vi "Digital Pulse Output.vi"() -> ()   [LabVIEW 2019]
uses:
  <vilib>/Utility/error.llb/DialogType.ctl
  <vilib>/DAQmx/configure/timing.llb/DAQmx Timing (Implicit).vi
  <vilib>/DAQmx/create/channels.llb/DAQmx Create Channel (CO-Pulse Generation-Frequency).vi
  <vilib>/DAQmx/read.llb/DAQmx Read (Counter 1D U32 1Chan NSamp).vi
  <vilib>/DAQmx/create/channels.llb/DAQmx Create Channel (CI-Count Edges).vi
panel:
  out "Waveform Chart":dynamicdata(graph)
  in  "stop (F) 2":bool caption="stop (F)"
  in  "stop (F)":bool
  in  "Stop":bool
  in  "counter":tag
  in  "counter 2":tag
  in  "Samples per Loop":i32=100
  in  "Stop 2":bool
  out "Data":u32[](array[numeric])
  in  "Duty Cycle":dbl=0.5 format="%.6f"
  in  "Frequency":dbl=1.0 format="%.6f"
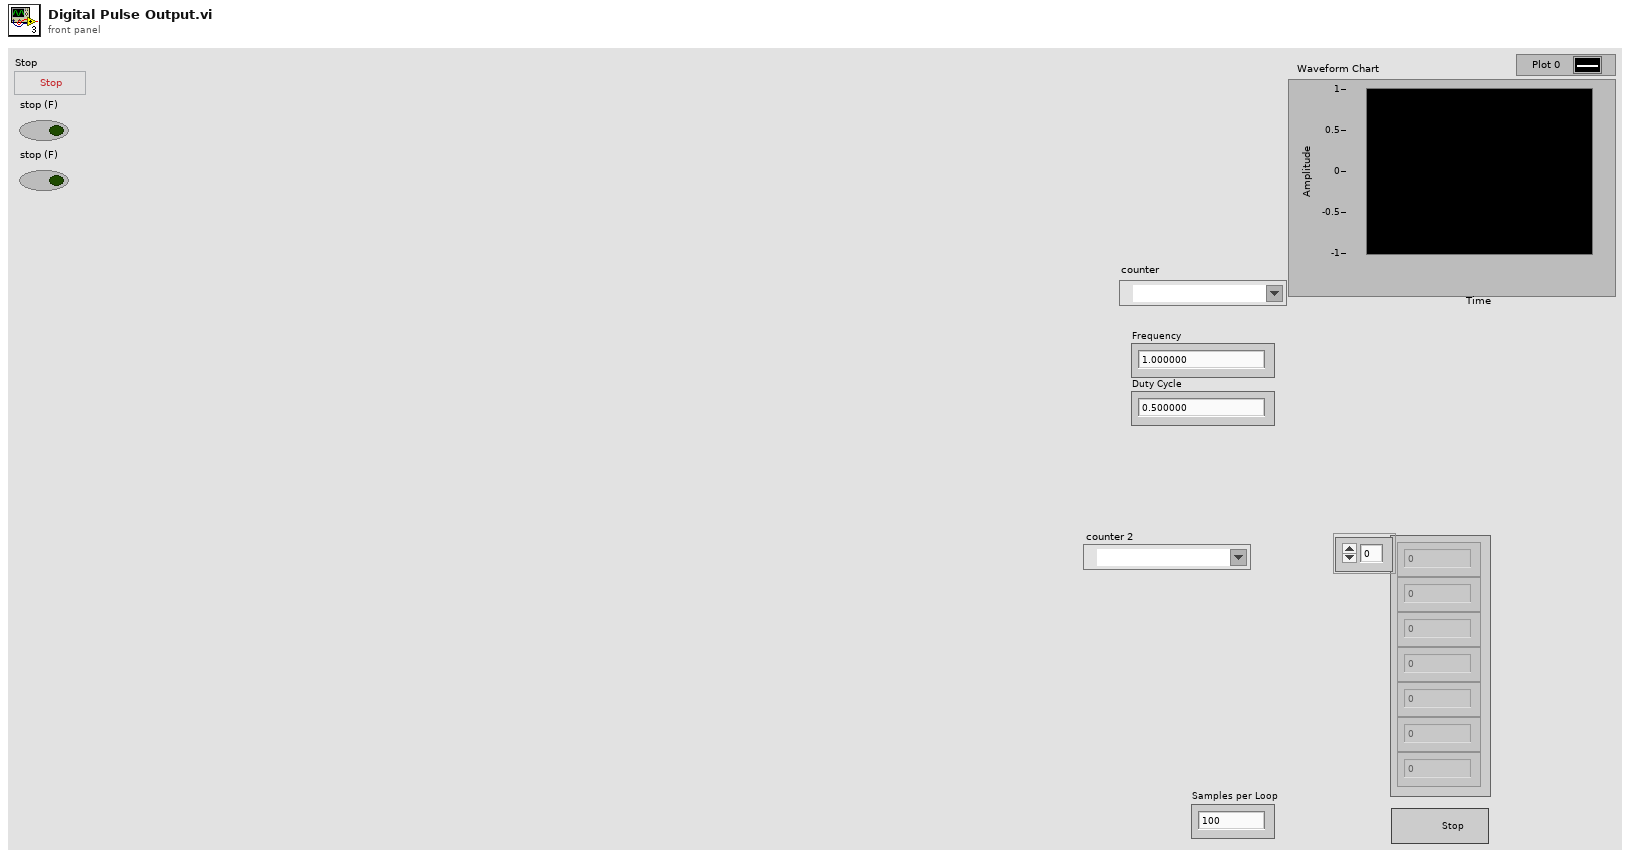
[diagram p1: front panel]
types:
  T1 = typedef "DialogType.ctl" = u16
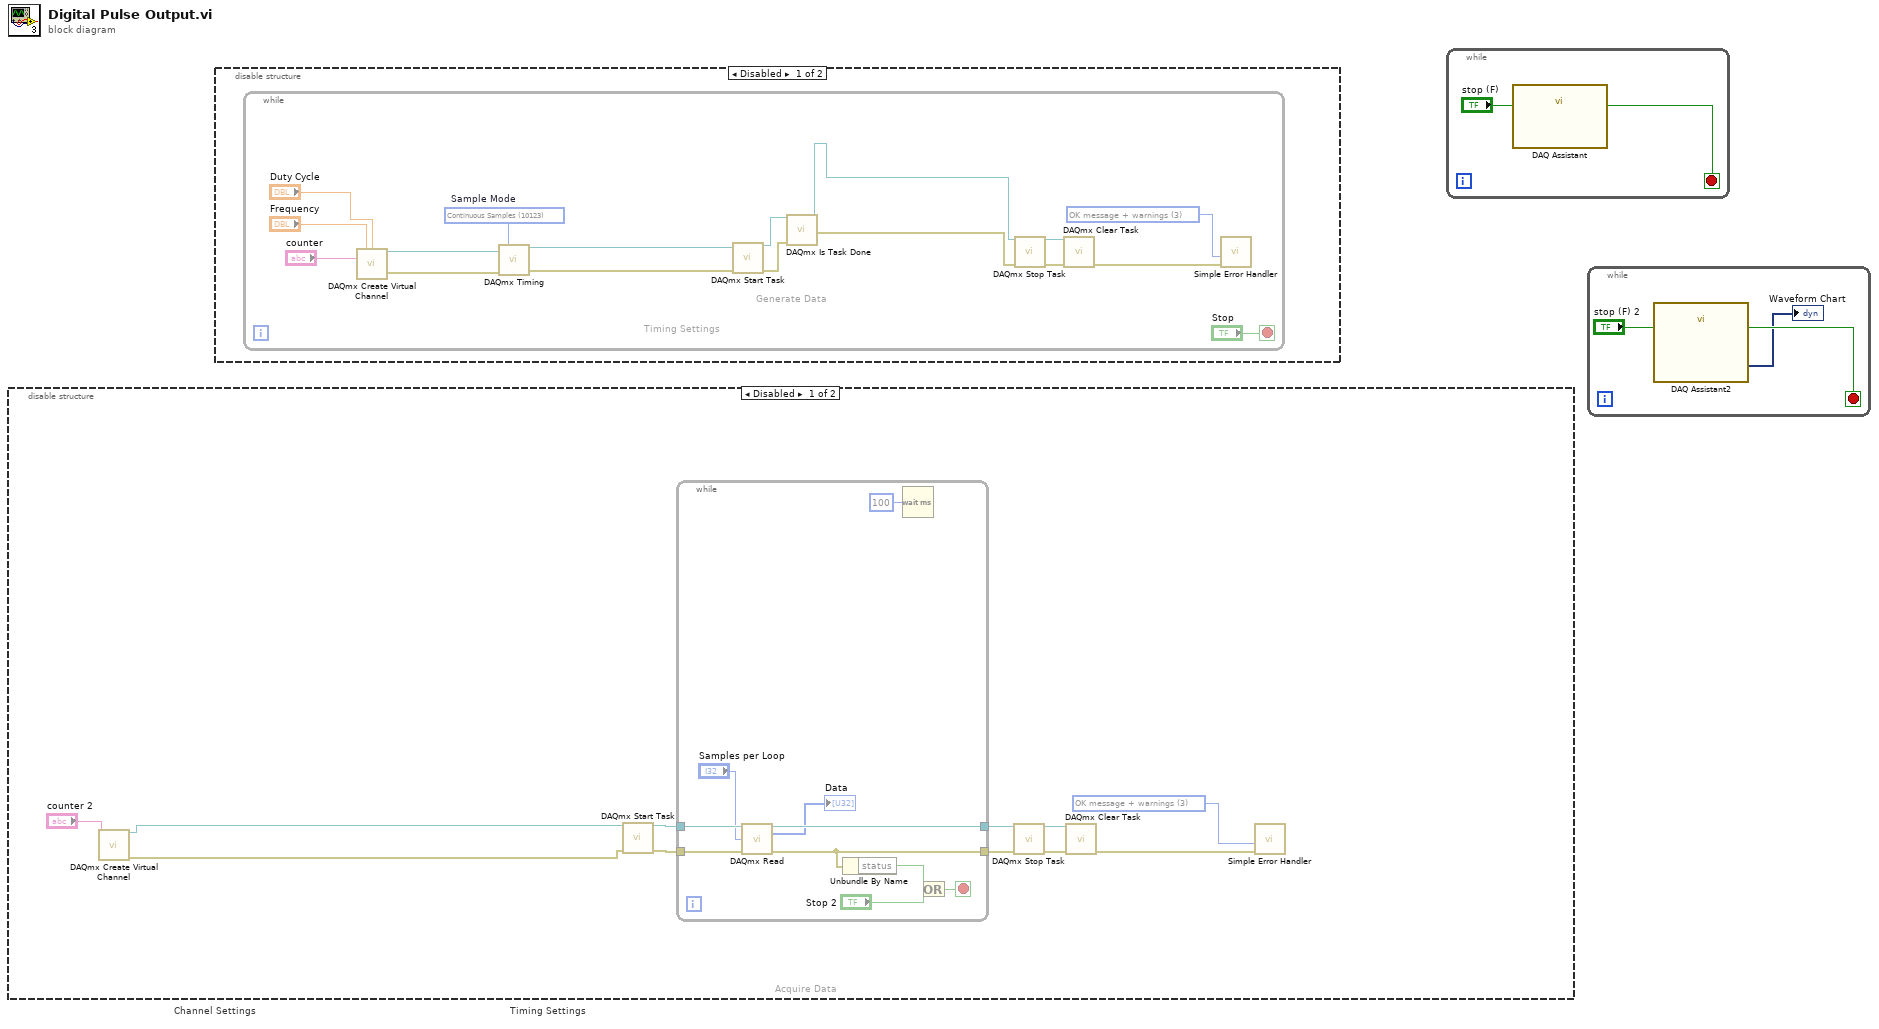
[diagram p0: block diagram]
diagram:
  # "Timing Settings"
  # "Channel Settings"
  n1 = disable-structure shown="Disabled" {
    frame Disabled {
      w4 = T1 3 items=["no dialog", "OK message", "continue or stop message", "OK message + warnings", "continue/stop + warnings"] ("type of dialog (OK msg:1)")
      # "Acquire Data"
      n2 = call-poly <vilib>:"DAQmx Create Virtual Channel.vi"("counter"="counter 2") -> ("task out"=w2:refnum<k21>, "error out"=w1:errorcluster)  [unwired: 13 in]
      n3 = call <vilib>:"DAQmx Start Task.vi"("task/channels in"=w2, "error in"=w1) -> ("task out"=w11:refnum<k21>, "error out"=w10:errorcluster)  [unwired: 12 in]
      n4 = while {
        tunnel: w11 -> [w21]
        tunnel: w10 -> [w20]
        tunnel: [w17] -> w7
        tunnel: [w18] -> w8
        stop <- w19 stop-if-true
        n5 = call-poly <vilib>:"DAQmx Read.vi"("task/channels in"=w21, "number of samples per channel"="Samples per Loop", "error in"=w20) -> ("task out"=w18:refnum<k21>, "data"=→"Data":u32[], "error out"=w17:errorcluster)  [unwired: 10 in]
        n6 = Unbundle By Name(w17) -> ("status"=w16:bool)
        n7 = Wait (ms)(milliseconds to wait=u32 100) -> ()  [unwired: 1 out]
        n8 = Or(x=w16, y="Stop 2") -> (x .or. y?=w19:bool)
      }
      n9 = call <vilib>:"DAQmx Stop Task.vi"("task/channels in"=w8, "error in"=w7) -> ("task out"=w5:refnum<k21>, "error out"=w6:errorcluster)  [unwired: 12 in]
      n10 = call <vilib>:"DAQmx Clear Task.vi"("task in"=w5, "error in"=w6) -> ("error out"=w9:errorcluster)  [unwired: 13 in]
      n11 = call <vilib>:"Simple Error Handler.vi"("type of dialog (OK msg:1)"=w4, "error in (no error)"=w9) -> ()  [unwired: 3 in, 5 out]
    }
    frame Enabled {
    }
  }
  n12 = disable-structure shown="Disabled" {
    frame Disabled {
      n13 = while {
        stop <- "Stop" stop-if-true
        w34 = T1 3 items=["no dialog", "OK message", "continue or stop message", "OK message + warnings", "continue/stop + warnings"] ("type of dialog (OK msg:1)")
        w38 = 10123 items=["Finite Samples"=10178, "Continuous Samples"=10123, "Hardware Timed Single Point"=12522]  # Sample Mode
        # "Generate Data"
        # "Timing Settings"
        n14 = call-poly <vilib>:"DAQmx Create Virtual Channel.vi"("frequency"="Frequency", "duty cycle"="Duty Cycle", "counter"="counter") -> ("task out"=w32:refnum<k21>, "error out"=w31:errorcluster)  [unwired: 11 in]
        n15 = call-poly <vilib>:"DAQmx Timing.vi"("task/channels in"=w32, "sample mode"=w38, "error in"=w31) -> ("task out"=w28:refnum<k21>, "error out"=w27:errorcluster)  [unwired: 11 in]
        n16 = call <vilib>:"DAQmx Start Task.vi"("task/channels in"=w28, "error in"=w27) -> ("task out"=w26:refnum<k21>, "error out"=w25:errorcluster)  [unwired: 12 in]
        n17 = call <vilib>:"DAQmx Is Task Done.vi"("task/channels in"=w26, "error in"=w25) -> ("task out"=w23:refnum<k21>, "error out"=w24:errorcluster)  [unwired: 11 in, 1 out]
        n18 = call <vilib>:"DAQmx Stop Task.vi"("task/channels in"=w23, "error in"=w24) -> ("task out"=w36:refnum<k21>, "error out"=w35:errorcluster)  [unwired: 12 in]
        n19 = call <vilib>:"DAQmx Clear Task.vi"("task in"=w36, "error in"=w35) -> ("error out"=w37:errorcluster)  [unwired: 13 in]
        n20 = call <vilib>:"Simple Error Handler.vi"("type of dialog (OK msg:1)"=w34, "error in (no error)"=w37) -> ()  [unwired: 3 in, 5 out]
      }
    }
    frame Enabled {
    }
  }
  n21 = while {
    stop <- w39 stop-if-true
    n22 = call "DAQ Assistant"("stop (F)"="stop (F)") -> ("stopped"=w39:bool)  [unwired: 16 in, 2 out]
  }
  n23 = while {
    stop <- w42 stop-if-true
    n24 = call "DAQ Assistant2"("stop (F)"="stop (F) 2") -> ("data"=→"Waveform Chart":dynamicdata, "stopped"=w42:bool)  [unwired: 15 in, 2 out]
  }
